vi "iDDS to FPGA.vi"(9 "Laser(V)":dbl[](array[numeric]), 11 "Chirp Parameters":T11) -> (1 "HEX Array":string[](array[string]), 3 "Interrupted":bool)   [LabVIEW 2020]
uses:
  Controls/Frequency Record.ctl
  Global Variables/General Globals.vi
  Controls/Pockels_Galvo_Params.ctl
  Typedefs/HW config states enum.ctl
  Typedefs/Chirp_ABCD.ctl
  Typedefs/XY Stage config cluster.ctl
  <vilib>/userDefined/High Color/nirio_resource_hc.ctl
  RIG-SPECIFIC FILES/FPGA Refs/FPGA Ref.ctl
  Typedefs/FPGA input type AC-DC.ctl
  Typedefs/DAQ FPGA config cluster.ctl
  Typedefs/DAQmx physical channels cluster.ctl
  Typedefs/CTRL system config cluster.ctl
  Typedefs/Encoder config cluster.ctl
  Typedefs/Cam VidRec HW config setup cluster.ctl
  Typedefs/Sys Configuration.ctl
panel:
  out "difftime - aodcontrol delay":dbl
  out "diff time":dbl
  in  "frontpanel":bool
  in  "System Config out":T1={"XY Stage"={"COM port"="", "XY stage available"=FALSE, "Baudrate"=0, "Type"=""}, "DAQ FPGA"={"Target"="RIO0", "input card type"=enum."AC Card", "Ref"=refnum, "Clock Freq (MHz) "=200.0, "Samples Wait after Trigger"=5080, "AOD fill"=4900, "StartupDelay"=0, "Slip Cycle (clock cycles)"=600000, "Add Cycle"=TRUE}, "Control system"={"Contrl Sys Available Ind"=FALSE, "Control system.FPGA Type"=enum."Virtex 7", "Control system.Network adapter name"="", "Control system.MAC address"="", "Control system.Ethernet Port"=0, "Ethernet opened"=FALSE, "Ctrl FPGA Clock (MHz)"=240.0, "AOD 1 Amplitude"=0, "AOD 2 Amplitude"=0, "AOD 3 Amplitude"=0, "AOD 4 Amplitude"=0, "AOD 5 Amplitude"=0, "AOD 6 Amplitude"=0, "Data Time Interval (ns)"=0.0, "T0 (ns)"=0.0, "Ta (ns)"=0.0}, "Encoder"={"IP address"="224.0.1.103", "Port"=7000, "Wheel radius (cm)"=16.0, "Encoder Trigger"=""}, "DAQmx Chan"={"Pockels AO"="", "Hard shutter AO"="", "PMT AOs"="", "Galvo AOs"="", "Power meter AI"=""}, "Computer MAC address"="", "Cam VidRec"={"DO flag-Video record"="", "DO flag-Trial start"=""}, "Externalise Triggers"=FALSE, "MC Supported"=FALSE, "Laser wavelength (nm)"=920.0} {"Laser wavelength (nm)" min=800.0 max=1080.0 step=1.0; "Encoder"."Wheel radius (cm)" format="%#_13g"; "Control system"."Control system.Ethernet Port" min=0 max=2048 step=1; "Control system"."Ctrl FPGA Clock (MHz)" min=80.0 max=500.0 step=1.0; "Control system"."Data Time Interval (ns)" min=0.0 max=2048.0 step=1.0; "Control system"."Ta (ns)" min=0.0 max=2048.0 step=1.0; "Control system"."T0 (ns)" min=0.0 max=2048.0 step=1.0; "Control system"."AOD 6 Amplitude" min=0 max=2048 step=1; "Control system"."AOD 5 Amplitude" min=0 max=2048 step=1; "Control system"."AOD 4 Amplitude" min=0 max=2048 step=1; "Control system"."AOD 3 Amplitude" min=0 max=2048 step=1; "Control system"."AOD 2 Amplitude" min=0 max=2048 step=1; "Control system"."AOD 1 Amplitude" min=0 max=2048 step=1}
  out "Loop index":i32
  # "RE-ENTRANT"
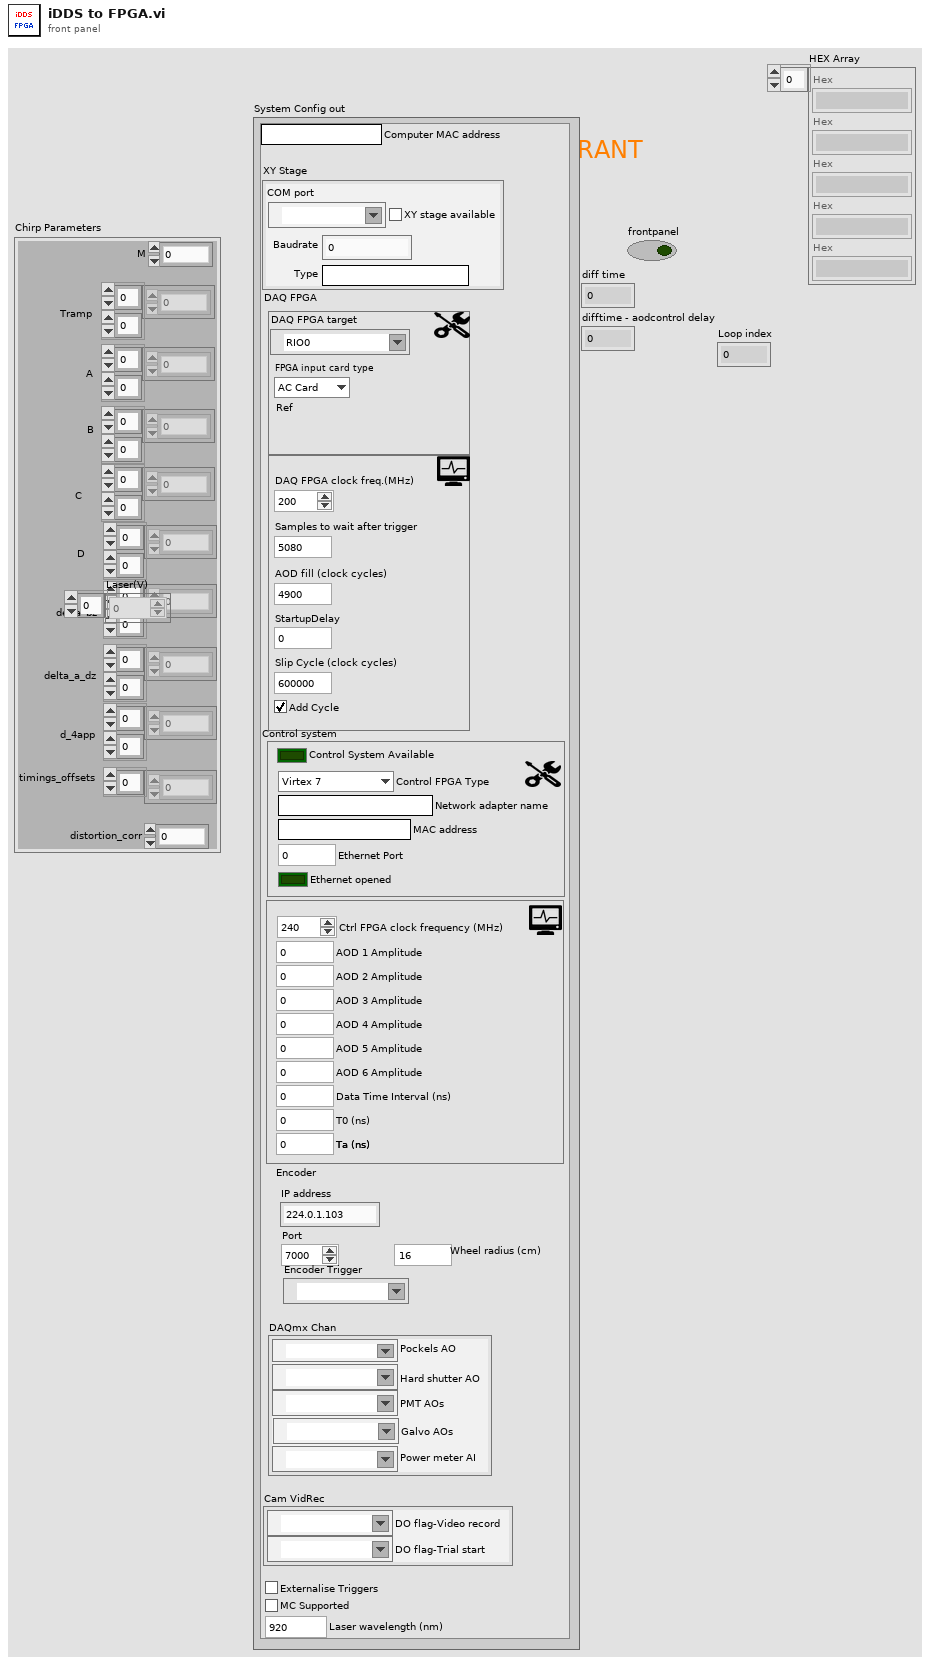
[diagram p1: front panel]
types:
  T1 = typedef "Sys Configuration.ctl" = cluster{"XY Stage":T2, "DAQ FPGA":T3, "Control system":T7, "Encoder":T8, "DAQmx Chan":T9, "Computer MAC address":string, "Cam VidRec":T10, "Externalise Triggers":bool, "MC Supported":bool, "Laser wavelength (nm)":dbl}
  T2 = typedef "XY Stage config cluster.ctl" = cluster{"COM port":refnum<visa-resource-name>, "XY stage available":bool, "Baudrate":i32, "Type":string}
  T3 = typedef "DAQ FPGA config cluster.ctl" = cluster{"Target":T4, "input card type":T5, "Ref":T6, "Clock Freq (MHz) ":dbl, "Samples Wait after Trigger":u16, "AOD fill":u16, "StartupDelay":i32, "Slip Cycle (clock cycles)":u32, "Add Cycle":bool}
  T4 = typedef "nirio_resource_hc.ctl" = tag
  T5 = typedef "FPGA input type AC-DC.ctl" = enum16{"AC Card", "DC Card"}
  T6 = typedef "FPGA Ref.ctl" = refnum<k20>
  T7 = typedef "CTRL system config cluster.ctl" = cluster{"Contrl Sys Available Ind":bool, "Control system.FPGA Type":enum16{"Virtex 5", "Virtex 7"}, "Control system.Network adapter name":string, "Control system.MAC address":string, "Control system.Ethernet Port":i16, "Ethernet opened":bool, "Ctrl FPGA Clock (MHz)":dbl, "AOD 1 Amplitude":i16, "AOD 2 Amplitude":i16, "AOD 3 Amplitude":i16, "AOD 4 Amplitude":i16, "AOD 5 Amplitude":i16, "AOD 6 Amplitude":i16, "Data Time Interval (ns)":dbl, "T0 (ns)":dbl, "Ta (ns)":dbl}
  T8 = typedef "Encoder config cluster.ctl" = cluster{"IP address":string, "Port":u16, "Wheel radius (cm)":dbl, "Encoder Trigger":tag}
  T9 = typedef "DAQmx physical channels cluster.ctl" = cluster{"Pockels AO":tag, "Hard shutter AO":tag, "PMT AOs":tag, "Galvo AOs":tag, "Power meter AI":tag}
  T10 = typedef "Cam VidRec HW config setup cluster.ctl" = cluster{"DO flag-Video record":tag, "DO flag-Trial start":tag}
  T11 = typedef "Chirp_ABCD.ctl" = cluster{"M ":dbl, "Tramp":dbl[][], "A":dbl[][], "B":dbl[][], "C":dbl[][], "D":dbl[][], "delta_bz":dbl[][], "delta_a_dz":dbl[][], "d_4app":dbl[][], "timings_offsets":dbl[], "distortion_corr":dbl}
  T12 = typedef "Pockels_Galvo_Params.ctl" = cluster{"A":dbl[], "Pockels Level":dbl[], "X Galvo":dbl[], "Y Galvo":dbl[], "AOD Fill Cycles":dbl[], "delta_a_dz":dbl[]}
  T13 = typedef "Frequency Record.ctl" = cluster{"Phi":dbl[], "A":dbl[], "B":dbl[], "C":dbl[], "D":dbl[], "E":dbl[], "Tstart":dbl[], "Tframe":dbl[]}
  T14 = cluster{"AOD 1 Amplitude":i16, "AOD 2 Amplitude":i16, "AOD 3 Amplitude":i16, "AOD 4 Amplitude":i16, "Center Frequency":dbl}
  T15 = typedef "HW config states enum.ctl" = enum16{"Load from file", "Save to file", "Save backup", "Write all", "Read all", "Write XY stage settings", "Write DAQ FPGA settings", "Write Control FPGA settings", "Write Phys Channels", "Write System Config", "Write HW Config", "Save System Config", "Save HW Config", "Clear", "Compare from file"}
  T16 = typedef "System Configuration.ctl" = cluster{"Laser wavelength (nm)":dbl, "DAQ FPGA System":T17, "Control system":T18}
  T17 = typedef "DAQ FPGA system config.ctl" = cluster{"Clock Freq (MHz) ":dbl, "Samples Wait after Trigger":u16, "AOD fill":u16, "StartupDelay":i32, "Slip Cycle (clock cycles)":u32, "Add Cycle":bool}
  T18 = typedef "CTRL system config.ctl" = cluster{"AOD 1 Amplitude":i16, "AOD 2 Amplitude":i16, "AOD 3 Amplitude":i16, "AOD 4 Amplitude":i16, "AOD 5 Amplitude":i16, "AOD 6 Amplitude":i16, "T0 (ns)":dbl, "Ta (ns)":dbl, "Data Time Interval (ns)":dbl, "Ctrl FPGA Clock (MHz)":dbl}
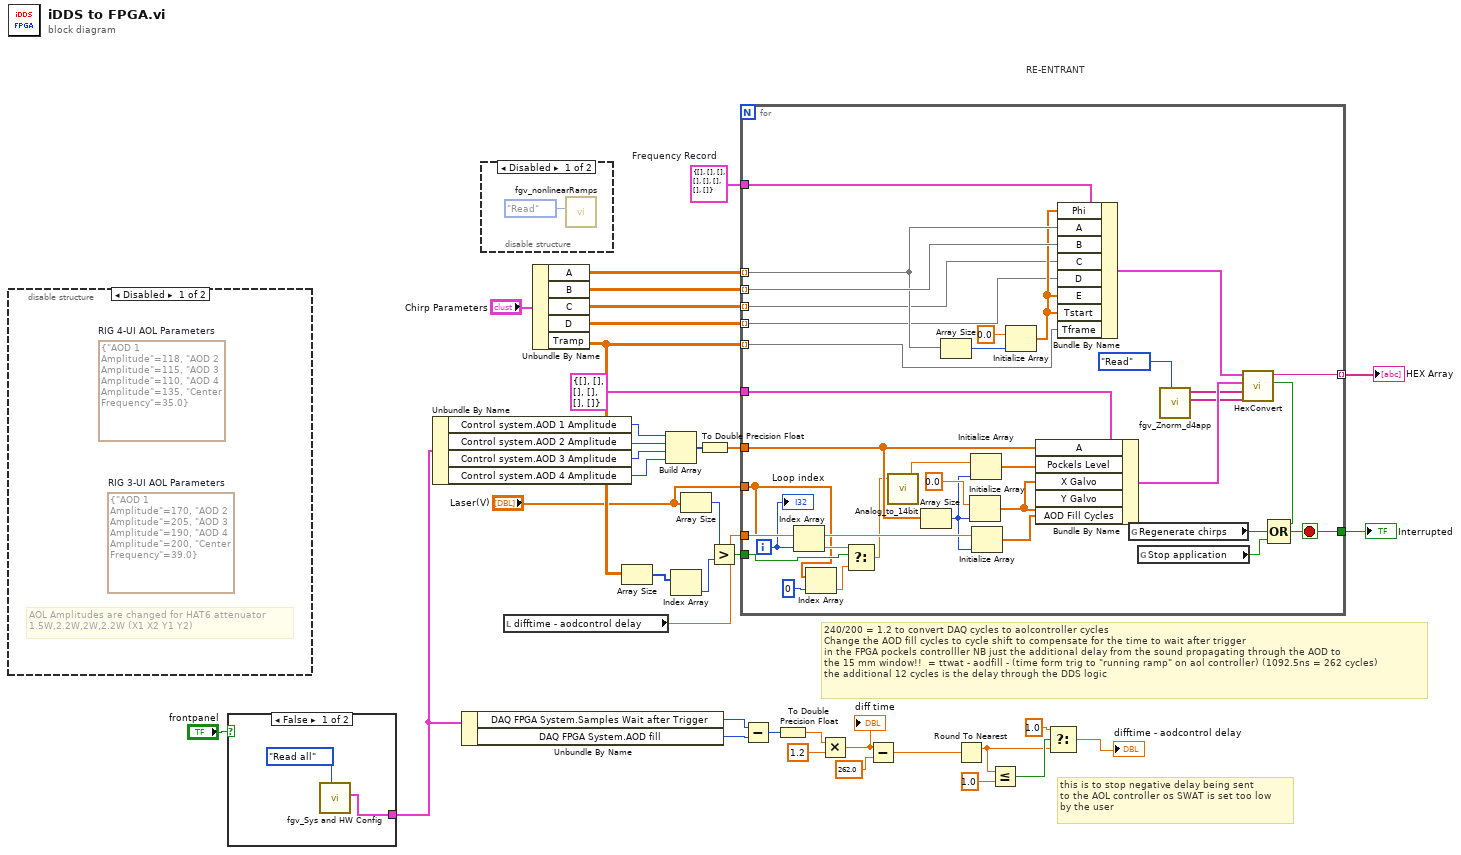
[diagram p0: block diagram]
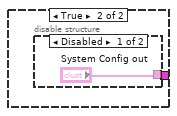
[diagram p2: hidden frame]
diagram:
  w37 = T13 {"Phi"=[], "A"=[], "B"=[], "C"=[], "D"=[], "E"=[], "Tstart"=[], "Tframe"=[]}  # Frequency Record
  # "this is to stop negative delay being sent\nto the AOL controller os SWAT is set too low\nby the user"
  # "240/200 = 1.2 to convert DAQ cycles to aolcontroller cycles\nChange the AOD fill cycles to cycle shift to compensate for the time to wait after trigger\nin the FPGA pockels controlller NB just the additional delay from the sound propagating through the AOD to\nthe 15 mm window!!  = ttwat - aodfill - (time form trig to \"running ramp\" on aol controller) (1092.5ns = 262 cycles)\nthe additional 12 cycles is the delay through the DDS logic"
  # "RE-ENTRANT"
  n1 = disable-structure shown="Disabled" {
    frame Disabled {
      (unwired) T14 {"AOD 1 Amplitude"=118, "AOD 2 Amplitude"=115, "AOD 3 Amplitude"=110, "AOD 4 Amplitude"=135, "Center Frequency"=35.0}  # RIG 4-UI AOL Parameters
      (unwired) T14 {"AOD 1 Amplitude"=170, "AOD 2 Amplitude"=205, "AOD 3 Amplitude"=190, "AOD 4 Amplitude"=200, "Center Frequency"=39.0}  # RIG 3-UI AOL Parameters
      # "AOL Amplitudes are changed for HAT6 attenuator\n1.5W,2.2W,2W,2.2W (X1 X2 Y1 Y2)"
    }
    frame Enabled {
    }
  }
  n2 = case shown="False" "frontpanel" {
    tunnel: [w38 _] -> w1
    frame False {
      n3 = call "fgv_Sys and HW Config.vi"("Function"=HW_config_states_enum."Read all") -> ("System Config OUT"=w38:T16)  [unwired: 8 in, 2 out]
    }
    frame True {
      n4 = disable-structure shown="Disabled" {
        disable-tunnel: ["System Config out" _] -> _
        frame Disabled {
        }
        frame Enabled {
        }
      }
    }
  }
  n5 = Unbundle By Name(w1) -> ("Control system.AOD 1 Amplitude"=w34:i16, "Control system.AOD 2 Amplitude"=w33:i16, "Control system.AOD 3 Amplitude"=w32:i16, "Control system.AOD 4 Amplitude"=w31:i16)
  n6 = Unbundle By Name(w1) -> ("DAQ FPGA System.Samples Wait after Trigger"=w15:u16, "DAQ FPGA System.AOD fill"=w14:u16)
  n7 = disable-structure shown="Disabled" {
    frame Disabled {
      n8 = call "fgv_nonlinearRamps.vi"("Status"=enum16{"Initialize", "Write", "Read"}."Read") -> ()  [unwired: 8 in, 3 out]
    }
    frame Enabled {
    }
  }
  n9 = local read "difftime - aodcontrol delay"() -> (w7:dbl)
  n10 = Unbundle By Name("Chirp Parameters") -> ("A"=w30:dbl[][], "B"=w27:dbl[][], "C"=w28:dbl[][], "D"=w26:dbl[][], "Tramp"=w21:dbl[][])
  n11 = Array Size(array=w21) -> (size(s)=w20:i32[])
  n12 = Build Array(w34, w33, w32, w31) -> (w29:i16[])
  n13 = Index Array(array=w20) -> (element=w18:i32)  [unwired: 1 in]
  n14 = Array Size(array="Laser(V)") -> (size(s)=w17:i32)
  n15 = To Double Precision Float(number=w29) -> (double precision float=w24:dbl[])
  n16 = Greater?(x=w17, y=w18) -> (0:w16:bool)
  n17 = for {
    tunnel: w30 -> [w69] mode=indexing
    tunnel: w37 -> [w73]
    tunnel: T12 {"A"=[], "Pockels Level"=[], "X Galvo"=[], "Y Galvo"=[], "AOD Fill Cycles"=[], "delta_a_dz"=[]} ("Pockels_Galvo_Params") -> [w72]
    tunnel: w24 -> [w51]
    tunnel: w28 -> [w60] mode=indexing
    tunnel: w27 -> [w70] mode=indexing
    tunnel: w26 -> [w59] mode=indexing
    tunnel: [w66] -> w35 mode=indexing
    tunnel: [w65] -> w25
    tunnel: w21 -> [w62] mode=indexing
    tunnel: w7 -> [w58]
    tunnel: "Laser(V)" -> [w45]
    tunnel: w16 -> [w48]
    i -> [w52]
    stop <- w65 stop-if-true
    n18 = Index Array(array=w45, index=w52) -> (element=w49:dbl)
    n19 = Index Array(array=w45, index=0) -> (element=w46:dbl)
    n20 = Select(t=w49, s=w48, f=w46) -> (s? t:f=w50:dbl)
    n21 = call "Analog_to_14bit.vi"("Pockels (0-2V)"=w50) -> ("Pockels Level(14 bit)"=w53:dbl)  [unwired: 10 in]
    n22 = Array Size(array=w51) -> (size(s)=w54:i32)
    n23 = Array Size(array=w69) -> (size(s)=w74:i32)
    n24 = Initialize Array(0.0 ("element"), w54) -> (w71:dbl[])
    n25 = Initialize Array(w53, w54) -> (w55:dbl[])
    n26 = Initialize Array(w58, w54) -> (w57:dbl[])
    n27 = Initialize Array(0.0 ("element"), w74) -> (w61:dbl[])
    n28 = Bundle By Name(cluster=w72, "A"=w51, "Pockels Level"=w55, "X Galvo"=w71, "Y Galvo"=w71, "AOD Fill Cycles"=w57) -> (w67:T12)
    n29 = Bundle By Name(cluster=w73, "Phi"=w61, "A"=w69, "B"=w70, "C"=w60, "D"=w59, "E"=w61, "Tstart"=w61, "Tframe"=w62) -> (w68:T13)
    n30 = global read "General Globals.vi" "Regenerate chirps"() -> (w65:bool)
    n31 = global read "General Globals.vi" "Stop application"() -> (w63:bool)
    n32 = call "fgv_Znorm_d4app.vi"("Function"=enum16{"Idle", "Write", "Read"}."Read") -> ("E Field"=w42:string[], "Phase Field"=w43:string[])  [unwired: 8 in, 1 out]
    n33 = call "HexConvert.vi"("E Field"=w42, "Phase Field"=w43, "Pockels_Galvo_Params"=w67, "Frequency Record"=w68) -> ("Interrupted"=w64:bool, "Hex"=w66:string)  [unwired: 6 in]
    n34 = Compound Arithmetic op=OR(w64, w65, w63) -> ()  [unwired: 1 out]
    "Loop index" <- w52
  }
  "HEX Array" <- w35
  "Interrupted" <- w25
  n35 = Subtract(x=w15, y=w14) -> (x-y=w13:u16)
  n36 = To Double Precision Float(number=w13) -> (double precision float=w12:dbl)
  n37 = Multiply(x=w12, y=1.2) -> (x*y=w10:dbl)
  "diff time" <- w10
  n38 = Subtract(x=w10, y=262.0) -> (x-y=w8:dbl)
  n39 = Round To Nearest(number=w8) -> (nearest integer value=w3:dbl)
  n40 = Less Or Equal?(x=w3, y=1.0) -> (x <= y?=w5:bool)
  n41 = Select(t=1.0, s=w5, f=w3) -> (s? t:f=→"difftime - aodcontrol delay":dbl)
